vi "Get Sampling Interval.vi"(8 "error in":errorcluster, 11 "Baseline Mocon \npiD-Tech plus in":refnum<class "Baseline Mocon piD-Tech plus.lvclass">) -> (0 "error out":errorcluster, 2 "Sampling Interval (ms)":u32=100, 3 "Baseline Mocon \npiD-Tech plus out":refnum<class "Baseline Mocon piD-Tech plus.lvclass">)   [LabVIEW 2011, in "Baseline Mocon piD-Tech plus.lvclass"]
uses:
  Baseline Mocon piD-Tech plus.lvclass
  Baseline Mocon piD-Tech plus.lvclass/Baseline Mocon piD-Tech plus.ctl
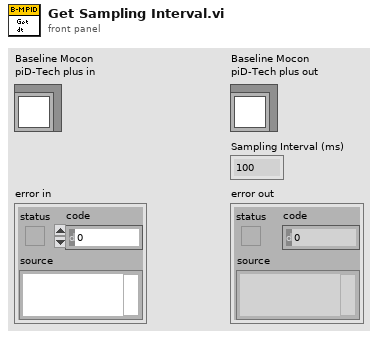
[diagram p1: front panel]
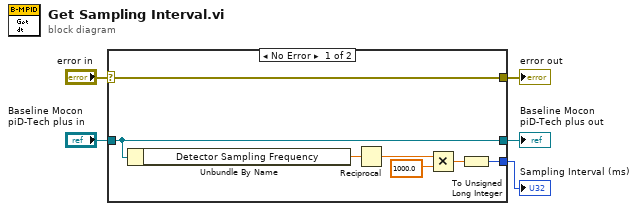
[diagram p0: block diagram]
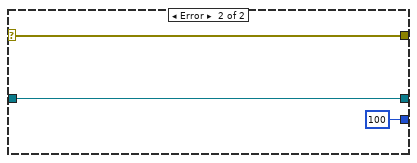
[diagram p2: hidden frame]
diagram:
  n1 = case shown="No Error" "error in" {
    selector: "error in" -> [w12 w15]
    tunnel: [w12 w15] -> w4
    tunnel: [w11 w14] -> w2
    tunnel: "Baseline Mocon \npiD-Tech plus in" -> [w11 w14]
    tunnel: [w9 u32 100] -> w1
    frame No Error {
      n2 = Unbundle By Name(w11) -> ("Detector Sampling Frequency"=w10:dbl)
      n3 = Reciprocal(x=w10) -> (1/x=w8:dbl)
      n4 = Multiply(x=w8, y=1000.0) -> (x*y=w6:dbl)
      n5 = To Unsigned Long Integer(number=w6) -> (unsigned 32bit integer=w9:u32)
    }
    frame Error {
    }
  }
  "error out" <- w4
  "Baseline Mocon \npiD-Tech plus out" <- w2
  "Sampling Interval (ms)" <- w1
